vi "PH_Beamline.color Exp LB BL.vi"(0 "i ref in":refnum<vi>, 2 "Color State Exp LB Input":i32, 5 "error in (no error)":errorcluster) -> (14 "i ref out":refnum<vi>, 19 "error out":errorcluster)   [LabVIEW 2014, in "PH_Beamline.lvlib"]
doc: "This Vi colors the Experiment Laserbay beamline elements."
uses:
  PH_Beamline.lvlib
  PH_Basics/PH_StatusHandler/PH_StatusHandler.Status.ctl
  PH_Basics/PH_Common/PH_Common.lvlib
  PH_BL-Master/PH_BL-Master.lvlib
  PH_Basics/PH_StatusHandler/PH_StatusHandler.lvlib
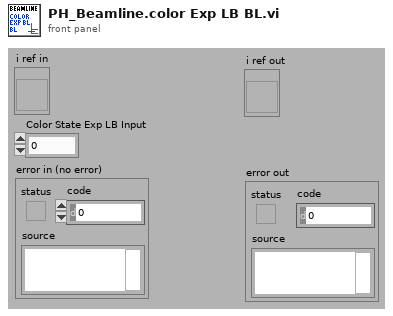
[diagram p1: front panel]
types:
  T1 = typedef "PH_StatusHandler.lvlib/PH_StatusHandler.Status.ctl" = i16
  T2 = typedef "PH_Beamline.lvlib/PH_Beamline.i attribute.ctl" = cluster{"GUI Refs":cluster{"PA ok":refnum<vi>, "MA ok":refnum<vi>, "fs FE ok":refnum<vi>, "ns FE ok":refnum<vi>, "PA ED ok":refnum<vi>, "MAS ok":refnum<vi>, "Booster ok":refnum<vi>, "Mirrortower ok":refnum<vi>, "In.-Box ok":refnum<vi>, "Compressor ok":refnum<vi>, "Experiment LB ok":refnum<vi>, "Experiment LL ok":refnum<vi>, "PHELIX_Beckhoff_Watchdog":refnum<vi>, "Shutters closed":refnum<vi>, "uOPA ok":refnum<vi>, "Vacuum no shotcond Comp LB":refnum<vi>}, "Refs BL MA":refnum<vi>[], "Refs BL MA-IB":refnum<vi>[], "Refs BL fs":refnum<vi>[], "Refs BL PA ED":refnum<vi>[], "Refs BL MAS":refnum<vi>[], "Refs BL Boo":refnum<vi>[], "Refs BL ns":refnum<vi>[], "Refs BL Mirrortower":refnum<vi>[], "Refs BL Compressor":refnum<vi>[], "Refs BL Exp LB":refnum<vi>[], "Radiation Safety":cluster{"Exp Laserbay":cluster{"Ref Op Mode":refnum<vi>, "Ref Laserbay evacuated":refnum<vi>, "Tagname LB evacuated":string, "Shot Mode":T3, "Laserbay evacuated?":i32, "Tagname HV room locked":string, "HV room locked?":i32, "Ref HV room locked":refnum<vi>, "Tagname bridged?":string, "Ref Bridge":refnum<vi>, "I<1E18W/cm²":bool}, "Exp Laserlab":cluster{"Ref Op Mode":refnum<vi>, "Ref Laserlab evacuated":refnum<vi>, "Tagname LL evacuated":string, "Shot Mode":T3, "Laserlab evacuated?":i32, "Tagname bridged?":string, "Ref Bridge":refnum<vi>, "I<1E18W/cm²":bool}}, "Refs BL LL":refnum<vi>[], "PP Igni Heating GUI Refs":refnum<vi>[], "PP Igni Heating Tagnames ":string[], "Refs BL PA":cluster{"undelayed Line before Shutter":refnum<vi>[], "undelayed Line after Shutter":refnum<vi>[], "before Bypass":refnum<vi>[], "delayed Line before Shutter":refnum<vi>[], "delayed Line after Shutter":refnum<vi>[], "before Shutter Input":refnum<vi>[], "after Shutter Input":refnum<vi>[], "Bypass":refnum<vi>[], "before Shutter Exit":refnum<vi>[], "after Shutter Exit":refnum<vi>[], "to MA":refnum<vi>[], "to Lab":refnum<vi>[]}, "BL":cluster{"YLF_BL_Status":i32, "fs_BL_Status":i32, "fs_YLF_BL_Status":i32, "ns_BL_Status":i32, "PA_Input_BL_Status":i32, "PA_UnDelay_BL_Status":i32, "PA_Delay_BL_Status":i32, "PA_BL_Status":i32, "PA_Bypass_BL_Status":i32, "PA_Exit_BL_Status":i32, "PA_LL_BL_Status":i32, "LL_BL_Status":i32, "PA_MA_BL_Status":i32, "MA_Exit_BL_Status":i32, "MA_Z6_BL_Status":i32, "Z6_BL_Status":i32, "MA_LB_BL_Status":i32, "LB_TB2_BL_Status":i32, "PA_before_Bypass_BL_Status":i32, "LB_TB3_BL_Status":i32}, "State Subsystems":cluster{"PA":bool, "MA":bool, "ns FE":bool, "fs FE":bool, "PA ED":bool, "In.-Box":bool, "MAS":bool, "Booster":bool, "Mirrortower":bool, "Compressor":bool, "Experiment LB":bool, "Experiment LL":bool, "uOPA":bool}, "Status Subscriber Information":T4, "Refs BL uOPA":refnum<vi>[], "PA_Input_2_Beam_6PWpGUI not linked?":bool, "PA_Input_Delay_6PGUI not linked?":bool, "Settings":T7}
  T3 = typedef "PH_Beamline.lvlib/PH_Beamline.Operation Mode.ctl" = i32
  T4 = typedef "PH_Beamline.lvlib/PH_Beamline.Status Subscriber Information.ctl" = cluster{"fs Swich YLF":T5, "fs Exit Shutter":T5, "ns Exit Shutter":T5, "PA Input Shutter":T5, "PA PC WP":T5, "PA PC WP 2":T5, "PA Bypass In":T5, "PA Bypass Out":T5, "PA CH 1":T5, "PA delayed":T5, "PA non delayed":T5, "PA Exit Shutter":T5, "PA Switch Lab":T5, "PA Bridge CH Input MA":T5, "MA Diffusor IB":T5, "MA IB Ready":T5, "MA CH 1":T5, "MA CH 2":T5, "MA CH 3":T5, "MA CH 4":T5, "MA Shutter Align Cam":T5, "MA Position MM5":T5, "Calorimeter Switch":T5, "BL Z6 CH 9":T5, "BL Z6 Beamdump":T5, "BL Z6 Shutter":T5, "COS Sensitivity Switch":T5, "Exp LB Shutter":T5, "Exp LB TB 2":T5, "Exp LB TB 3":T5, "PA LL Input CH":T5, "PA LL Output CH":T5, "LL Comp Input Shutter":T5, "LL Comp Output Shutter":T5, "LL Comp FF Shutter":T5, "Exp LL Shutter":T5, "MA IM In IB":T5, "MA IM Out IB":T5, "MA DB In IB":T5, "MA DB Out IB":T5, "Exp LB Shutter Interlock":T5, "Exp LL Shutter Interlock":T5, "MM1 Force Sensor":T5}
  T5 = typedef "PH_BL-Master.lvlib/PH_BL-Master.Status Subscriber Information.ctl" = cluster{"Index of element":i32, "Attributeset":T6}
  T6 = typedef "PH_BL-Master.lvlib/PH_BL-Master.Attribute Set.ctl" = enum16{"Boolean Status Service Subscriber", "Picture Status Service Subscriber"}
  T7 = typedef "PH_Beamline_Chief.lvlib/PH_Beamline_Chief.Settings.ctl" = cluster{"PA Doublepass Mode":bool, "Compressor Vaccuum LB not relevant":bool, "Windowshutter TB2 not relevant":bool, "Windowshutter TB3 not relevant":bool}
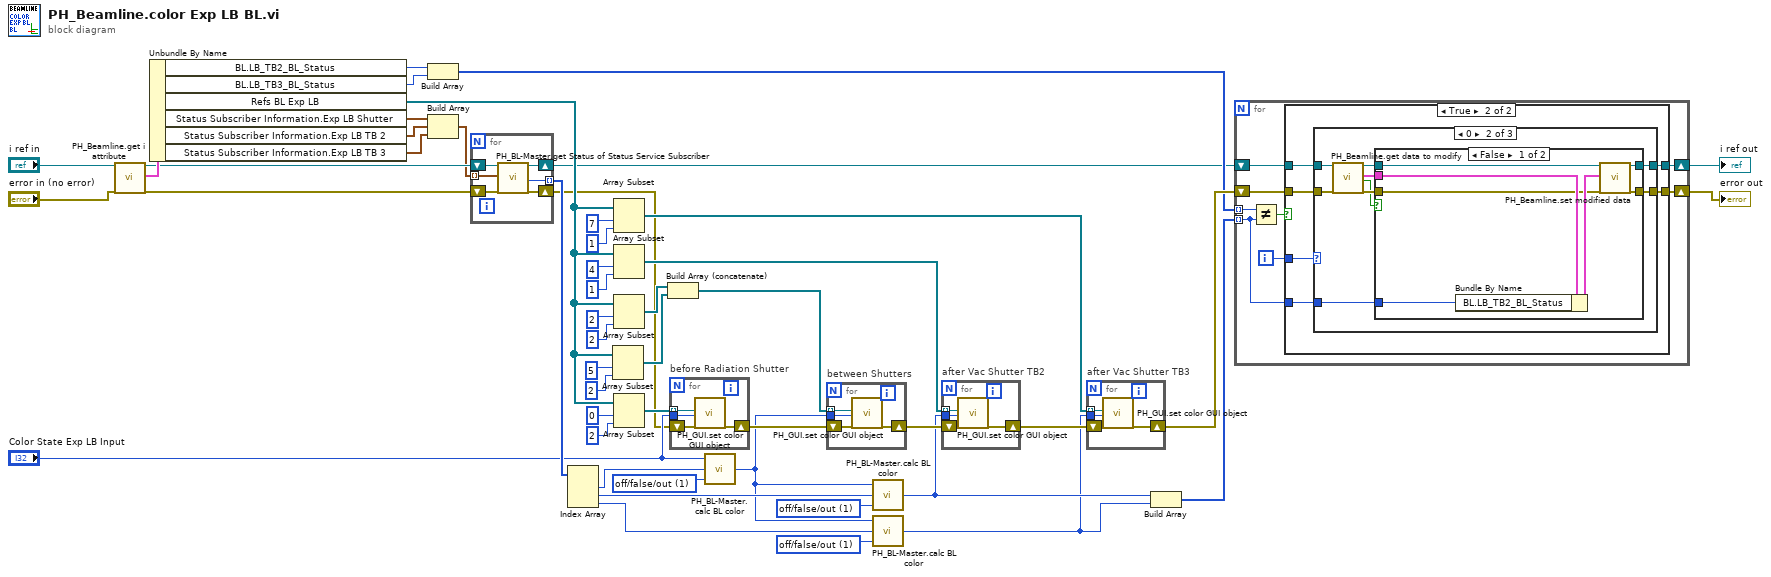
[diagram p0: block diagram]
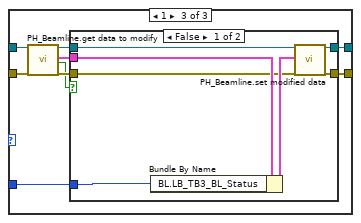
[diagram p5: hidden frame]
diagram:
  w16 = T1 1 items=["no info", "off/false/out", "on/true/in", "Failure", "Alarm", "Status 1", "Status 2", "Status 3"] ("State for \"2\" (on) of ABLE (off/false/out)")
  w33 = T1 1 items=["no info", "off/false/out", "on/true/in", "Failure", "Alarm", "Status 1", "Status 2", "Status 3"] ("State for \"2\" (on) of ABLE (off/false/out)")
  w34 = T1 1 items=["no info", "off/false/out", "on/true/in", "Failure", "Alarm", "Status 1", "Status 2", "Status 3"] ("State for \"2\" (on) of ABLE (off/false/out)")
  n1 = call "PH_Beamline.get i attribute.vi"("i ref in"="i ref in", "error in (no error)"="error in (no error)") -> ("i ref out"=w8:refnum<vi>, "i attribute"=w49:T2, "error out"=w7:errorcluster)  [unwired: 15 in]
  n2 = Unbundle By Name(w49) -> ("BL.LB_TB2_BL_Status"=w13:i32, "BL.LB_TB3_BL_Status"=w30:i32, "Refs BL Exp LB"=w21:refnum<vi>[], "Status Subscriber Information.Exp LB Shutter"=w4:T5, "Status Subscriber Information.Exp LB TB 2"=w3:T5, "Status Subscriber Information.Exp LB TB 3"=w2:T5)
  n3 = Build Array(w13, w30) -> (w14:i32[])
  n4 = Build Array(w4, w3, w2) -> (w1:T5[])
  n5 = for {
    tunnel: [w55] -> w38 mode=indexing
    tunnel: w1 -> [w50] mode=indexing
    shift-right: [w53] -> w9
    shift-left: w8 -> [w52]
    shift-right: [w54] -> w10
    shift-left: w7 -> [w51]
    n6 = call "PH_BL-Master.get Status of Status Service Subscriber.vi"("i ref in"=w52, "Wanted Status Subscriber Information"=w50, "error in (no error)"=w51) -> ("i ref out"=w53:refnum<vi>, "Status"=w55:T1, "error out"=w54:errorcluster)  [unwired: 11 in, 3 out]
  }
  n7 = Index Array(array=w38) -> (element #1=w36:T1, element #2=w35:T1, element #3=w17:T1)  [unwired: 3 in]
  n8 = Array Subset(array=w21, index=5 ("length"), length=2) -> (w24:refnum<vi>[])
  n9 = Array Subset(array=w21, index=7 ("length"), length=1) -> (w20:refnum<vi>[])
  n10 = Array Subset(array=w21, index=4 ("length"), length=1) -> (w39:refnum<vi>[])
  n11 = Array Subset(array=w21, index=2 ("length"), length=2) -> (w26:refnum<vi>[])
  n12 = Array Subset(array=w21, index=0, length=2) -> (w48:refnum<vi>[])
  n13 = Build Array (concatenate)(w26, w24) -> (w25:refnum<vi>[])
  n14 = for "before Radiation Shutter" {
    tunnel: w48 -> [w59] mode=indexing
    shift-right: [w57] -> w40
    shift-left: w10 -> [w58]
    tunnel: "Color State Exp LB Input" -> [w56]
    n15 = call "PH_GUI.set color GUI object.vi"("GUI object Ref"=w59, "State"=w56, "error in (no error)"=w58) -> ("error out"=w57:errorcluster)  [unwired: 16 in]
  }
  n16 = call "PH_BL-Master.calc BL color.vi"("State for \"2\" (on) of ABLE (off/false/out)"=w34, "State ABLE"=w36, "State before ABLE"="Color State Exp LB Input") -> ("State after ABLE"=w15:i32)
  n17 = for "between Shutters" {
    tunnel: w25 -> [w63] mode=indexing
    shift-right: [w61] -> w41
    shift-left: w40 -> [w62]
    tunnel: w15 -> [w60]
    n18 = call "PH_GUI.set color GUI object.vi"("GUI object Ref"=w63, "State"=w60, "error in (no error)"=w62) -> ("error out"=w61:errorcluster)  [unwired: 16 in]
  }
  n19 = call "PH_BL-Master.calc BL color.vi"("State for \"2\" (on) of ABLE (off/false/out)"=w33, "State ABLE"=w35, "State before ABLE"=w15) -> ("State after ABLE"=w29:i32)
  n20 = call "PH_BL-Master.calc BL color.vi"("State for \"2\" (on) of ABLE (off/false/out)"=w16, "State ABLE"=w17, "State before ABLE"=w15) -> ("State after ABLE"=w11:i32)
  n21 = for "after Vac Shutter TB2" {
    tunnel: w39 -> [w67] mode=indexing
    shift-right: [w65] -> w19
    shift-left: w41 -> [w66]
    tunnel: w29 -> [w64]
    n22 = call "PH_GUI.set color GUI object.vi"("GUI object Ref"=w67, "State"=w64, "error in (no error)"=w66) -> ("error out"=w65:errorcluster)  [unwired: 16 in]
  }
  n23 = for "after Vac Shutter TB3" {
    tunnel: w20 -> [w71] mode=indexing
    shift-right: [w69] -> w18
    shift-left: w19 -> [w70]
    tunnel: w11 -> [w68]
    n24 = call "PH_GUI.set color GUI object.vi"("GUI object Ref"=w71, "State"=w68, "error in (no error)"=w70) -> ("error out"=w69:errorcluster)  [unwired: 16 in]
  }
  n25 = Build Array(w29, w11) -> (w12:i32[])
  n26 = for {
    tunnel: w14 -> [w75] mode=indexing
    tunnel: w12 -> [w74] mode=indexing
    shift-right: [w76] -> w31
    shift-left: w18 -> [w73]
    shift-right: [w77] -> w32
    shift-left: w9 -> [w78]
    i -> [w72]
    n27 = Not Equal?(x=w75, y=w74) -> (x != y?=w79:bool)
    n28 = case shown="True" w79 {
      tunnel: w78 -> [w81 w87]
      tunnel: [w81 w86] -> w77
      tunnel: w73 -> [w80 w85]
      tunnel: [w80 w84] -> w76
      tunnel: w74 -> [_ w83]
      tunnel: w72 -> [_ w82]
      frame False {
      }
      frame True {
        n29 = case shown="0" w82 {
          tunnel: w87 -> [w89 w94 w112]
          tunnel: [w89 w93 w111] -> w86
          tunnel: w85 -> [w88 w92 w110]
          tunnel: [w88 w91 w109] -> w84
          tunnel: w83 -> [_ w90 w108]
          frame Default {
          }
          frame 0 {
            n30 = call "PH_Beamline.get data to modify.vi"("i ref in"=w94, "error in (no error)"=w92) -> ("i ref out"=w97:refnum<vi>, "i attribute"=w95:T2, "timed out"=w96:bool, "error out"=w98:errorcluster)  [unwired: 14 in]
            n31 = case shown="False" w96 {
              tunnel: w98 -> [w99 w106]
              tunnel: w97 -> [w105 w107]
              tunnel: [w104 w106] -> w91
              tunnel: [w103 w107] -> w93
              tunnel: w95 -> [w100 _]
              tunnel: w90 -> [w101 _]
              frame False {
                n32 = Bundle By Name(cluster=w100, "BL.LB_TB2_BL_Status"=w101) -> (w102:T2)
                n33 = call "PH_Beamline.set modified data.vi"("i ref in"=w105, "i attribute"=w102, "error in (no error)"=w99) -> ("i ref out"=w103:refnum<vi>, "error out"=w104:errorcluster)  [unwired: 15 in]
              }
              frame True {
              }
            }
          }
          frame 1 {
            n34 = call "PH_Beamline.get data to modify.vi"("i ref in"=w112, "error in (no error)"=w110) -> ("i ref out"=w115:refnum<vi>, "i attribute"=w113:T2, "timed out"=w114:bool, "error out"=w116:errorcluster)  [unwired: 14 in]
            n35 = case shown="False" w114 {
              tunnel: w116 -> [w117 w124]
              tunnel: w115 -> [w123 w125]
              tunnel: [w122 w124] -> w109
              tunnel: [w121 w125] -> w111
              tunnel: w113 -> [w118 _]
              tunnel: w108 -> [w119 _]
              frame False {
                n36 = Bundle By Name(cluster=w118, "BL.LB_TB3_BL_Status"=w119) -> (w120:T2)
                n37 = call "PH_Beamline.set modified data.vi"("i ref in"=w123, "i attribute"=w120, "error in (no error)"=w117) -> ("i ref out"=w121:refnum<vi>, "error out"=w122:errorcluster)  [unwired: 15 in]
              }
              frame True {
              }
            }
          }
        }
      }
    }
  }
  "error out" <- w31
  "i ref out" <- w32
